vi "CameraSerialPrototype_111.vi"() -> (4 "图像时间戳":u32=16532020 format="%_32g")   [LabVIEW 2015]
uses:
  <vilib>/Instr/_visa.llb/VISA Configure Serial Port (Instr).vi
  MVCAMSDK.dll
  <vilib>/Analysis/NI_AALBase.lvlib
panel:
  out "实时循环时间":u32
  in  "曝光时间":i32=50
  out "平移信号曲线":cluster{"Locations":dbl[], "Amplitudes":dbl[]}[](graph)=[{"Locations"=array[750 elements], "Amplitudes"=array[749 elements]}, {"Locations"=[104.38621227921368, 258.3247060234782, 410.71523318402836, 562.6858730022967, 712.7065754646931], "Amplitudes"=[11153.698204083417, 10559.387052180104, 10974.865031894917, 10500.852817232146, 11059.763900010517]}, {"Locations"=[26.787398227992274, 182.39455189327623, 333.5517219531509, 488.1851999460032, 636.5270621135614], "Amplitudes"=[3284.809720018355, 2039.4564261182056, 3638.2587716464914, 3082.2730888167225, 4217.856016996603]}]
  out "variance 2":dbl caption="方差" format="%0.2f"
  out "光强图 2":dbl[](graph)
  out "variance":dbl caption="方差" format="%0.2f"
  out "光强图":dbl[](graph)
  in  "平移前进":T1=TRUE
  in  "平移计数":u16
  in  "平移一次脉冲数":u16=20
  out "连接的字符串":string
  in  "flow control (0:none)":u16(ring) caption="流控制（0:无）" items=["无", "XON/XOFF", "RTS/CTS", "XON/XOFF & RTS/CTS", "DTR/DSR", "XON/XOFF & DTR/DSR"]
  in  "stop bits (10: 1 bit)":u16=10 caption="停止位（10: 1位）"
  in  "奇偶 (0:none)":enum16{"None", "Odd", "Even", "Mark", "Space"}(ring) caption="奇偶（0:无）"
  in  "数据比特(默认8)":u16(ring)=8 items=["5"=5, "6"=6, "7"=7, "8"=8]
  in  "波特率(默认9600)":u32=9600
  in  "端口":refnum<visa-resource-name>="COM1"
  in  "停止":bool
  out "帧速":u32
  out "帧间耗时\n单位：（0.1ms）":u32
  out "Image":T2(plugin-control)
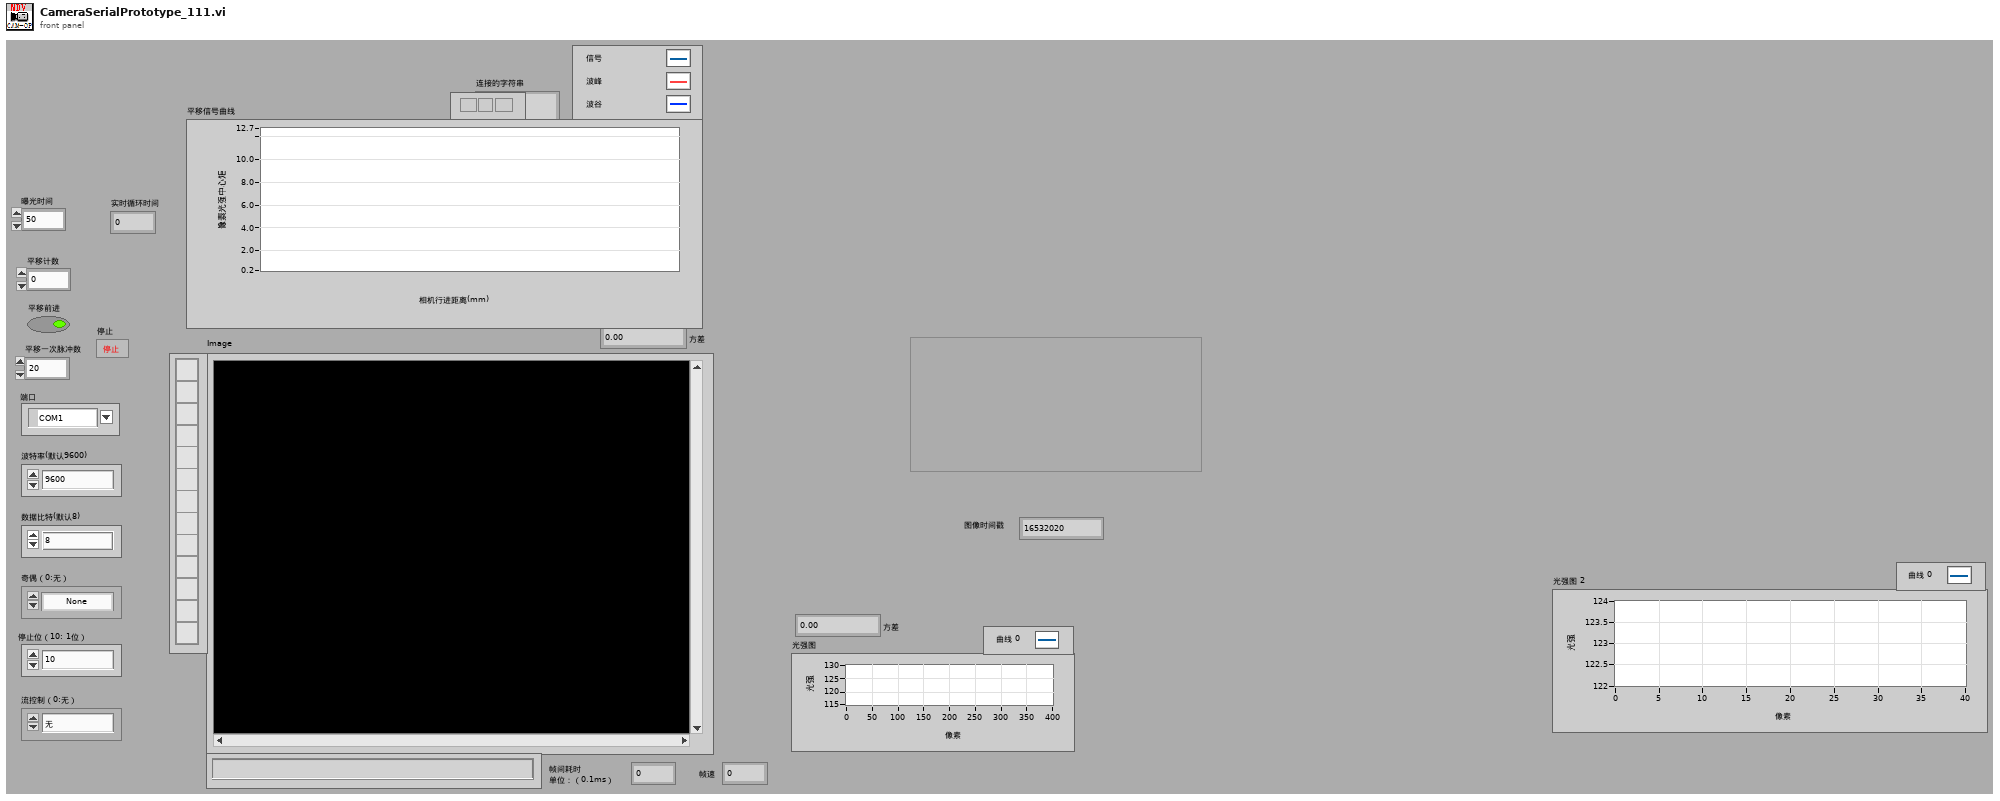
[diagram p1: front panel]
types:
  T1 = typedef "控件 1.ctl" = bool
  T2 = typedef "IMAQ Image.ctl" = refnum<image>
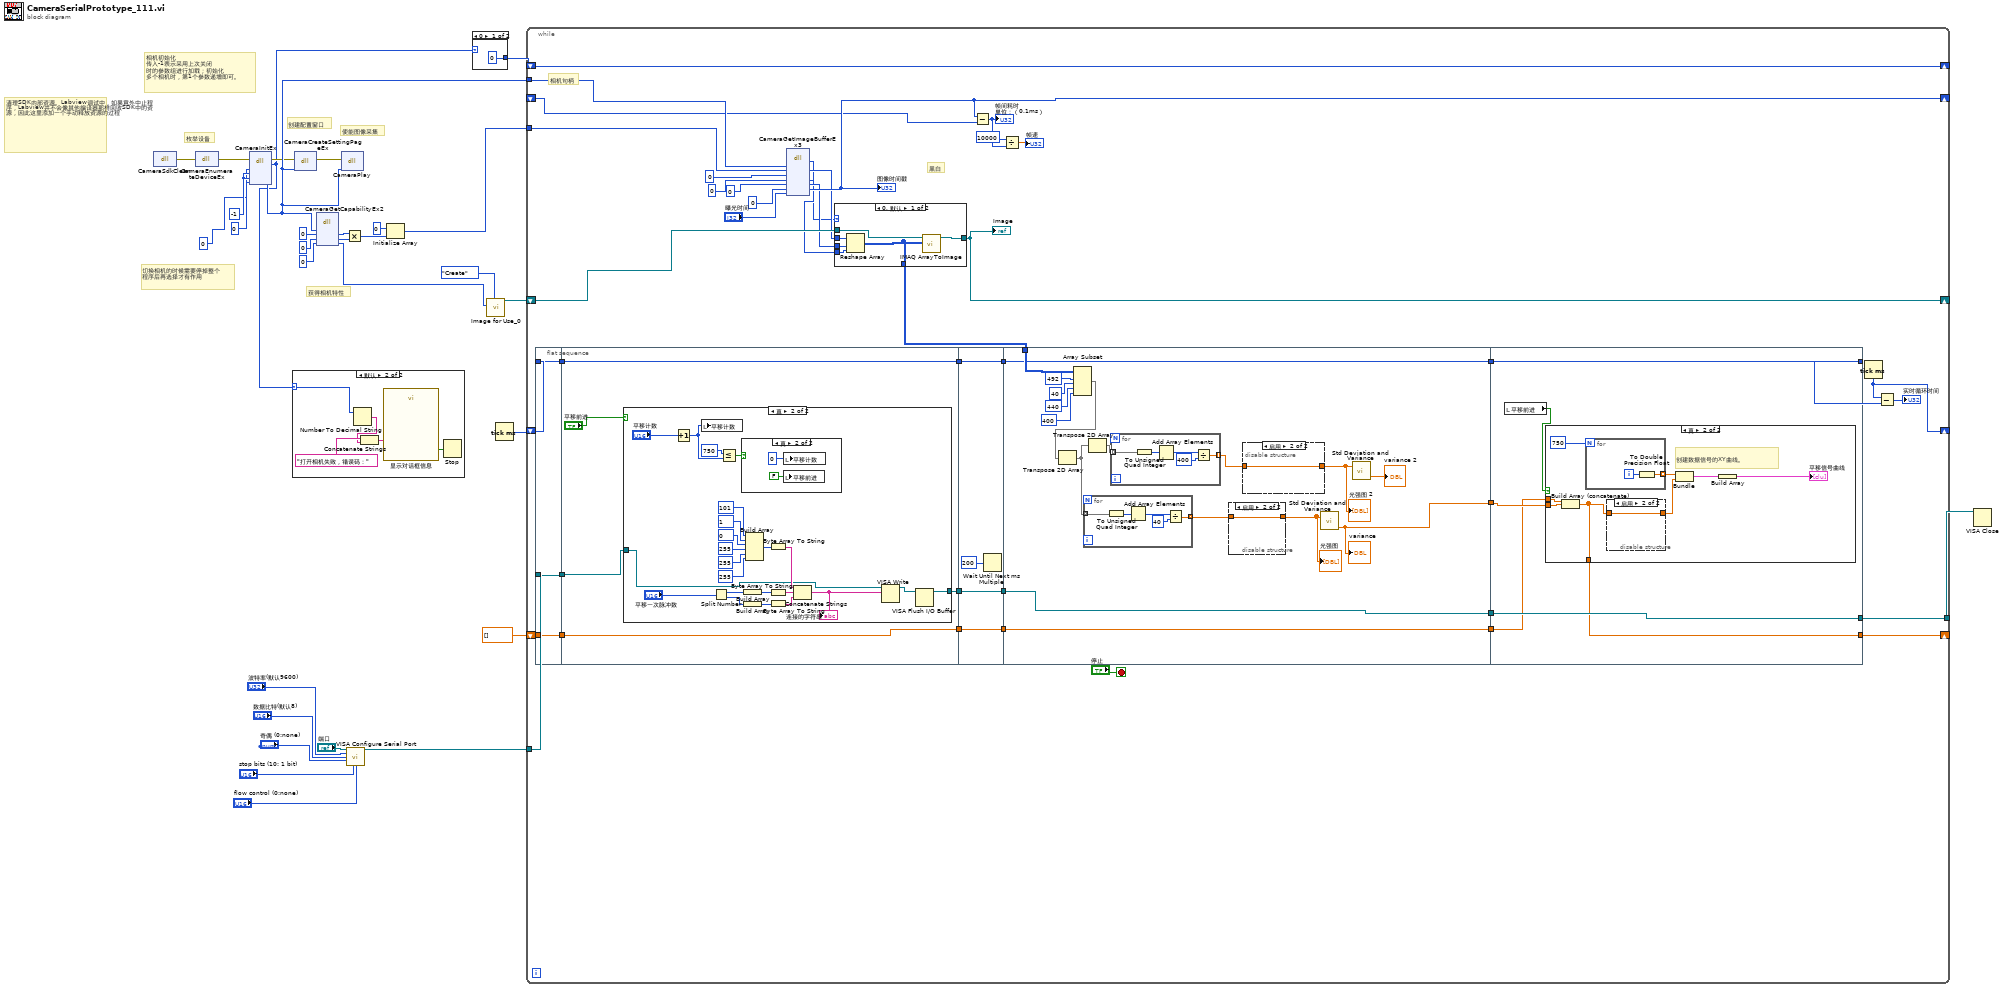
[diagram p0: block diagram]
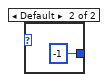
[diagram p2: hidden frame]
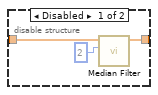
[diagram p6: hidden frame]
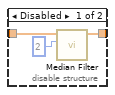
[diagram p7: hidden frame]
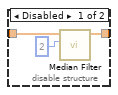
[diagram p9: hidden frame]
diagram:
  w29 = -1
  # "切换相机的时候需要停掉整个\n程序后再选择才有作用"
  # "清理SDK内部资源。Labview调试中，如果意外中止程序，Labview并不会像其他编译器那样回收SDK中的资源，因此这里添加一个手动释放资源的过程"
  # "使能图像采集"
  # "获得相机特性"
  # "创建配置窗口"
  # "相机初始化\n传入-1表示采用上次关闭\n时的参数组进行加载；初始化\n多个相机时，第1个参数递增即可。"
  # "枚举设备"
  n1 = dll-call lib="MVCAMSDK.dll" fn="CameraSdkClean"() -> (error out=w30:errorcluster)  [unwired: 4 in, 1 out]
  n2 = dll-call lib="MVCAMSDK.dll" fn="CameraEnumerateDeviceEx"(error in=w30) -> (error out=w27:errorcluster)  [unwired: 3 in, 1 out]
  n3 = dll-call lib="MVCAMSDK.dll" fn="CameraInitEx"(error in=w27, "相机索引值"=0, "参数加载方式"=w29, "要加载的参数组索引"=w29, "相机句柄"=0) -> (error out=w16:errorcluster, "返回类型"=w14:i32, "相机句柄"=w18:i32)  [unwired: 5 in, 1 out]
  n4 = case shown="默认" w14 {
    selector: w14 -> [_ w35]
    frame 0 {
    }
    frame Default {
      n5 = Number To Decimal String(number=w35) -> (decimal integer string=w32:string)  [unwired: 1 in]
      n6 = Concatenate Strings("打开相机失败，错误码：" ("字符串"), w32) -> (w34:string)
      n7 = call "显示对话框信息"("Message"=w34) -> ("结束"=w36:bool)  [unwired: 9 in, 1 out]
      n8 = Stop(stop? (T)=w36) -> ()
    }
  }
  n9 = dll-call lib="MVCAMSDK.dll" fn="CameraCreateSettingPageEx"(error in=w16, "相机句柄"=w18) -> (error out=w19:errorcluster)  [unwired: 4 in, 1 out]
  n10 = dll-call lib="MVCAMSDK.dll" fn="CameraGetCapabilityEx2"("相机句柄"=w18, "图像最大宽度"=0, "图像最大高度"=0, "是否是彩色相机(返回0:黑白;1:彩色)"=0) -> ("图像最大宽度"=w21:i32, "图像最大高度"=w20:i32, "是否是彩色相机(返回0:黑白;1:彩色)"=w12:i32)  [unwired: 5 in, 2 out]
  n11 = dll-call lib="MVCAMSDK.dll" fn="CameraPlay"(error in=w19, "相机句柄"=w18) -> ()  [unwired: 4 in, 2 out]
  n12 = Multiply(x=w21, y=w20) -> (x*y=w25:i32)
  n13 = call-poly "VISA Configure Serial Port"("VISA resource name"="端口", "baud rate (9600)"="波特率(默认9600)", "data bits (8)"="数据比特(默认8)", "parity (0:none)"="奇偶 (0:none)", "stop bits (10: 1 bit)"="stop bits (10: 1 bit)", "flow control (0:none)"="flow control (0:none)") -> ("VISA resource name out"=w4:refnum<visa-resource-name>)  [unwired: 8 in, 1 out]
  n14 = Initialize Array(0, w25) -> (w17:i32[])
  n15 = case shown="0" w14 {
    tunnel: [0 -1] -> w13
    frame 0 {
    }
    frame Default {
    }
  }
  n16 = call "Image for Use_0.vi"("Command"=enum16{"Create", "Use", "Copy in", "Dispose"}."Create", "Image Type"=w12) -> ("Image out"=w15:T2)  [unwired: 8 in, 1 out]
  n17 = Tick Count (ms)() -> (millisecond timer value=w1:u32)
  n18 = while {
    tunnel: w18 -> [w78]
    tunnel: w17 -> [w80]
    shift-right: [w77] -> _
    shift-left: w13 -> [w77]
    shift-right: [w76] -> _
    shift-left: w15 -> [w79]
    shift-right: [w75] -> _
    shift-left: _ -> [w74]
    tunnel: w4 -> [w53]
    tunnel: [w57] -> w3
    shift-right: [w54] -> _
    shift-left: dbl[] [] -> [w55]
    shift-right: [w49] -> _
    shift-left: w1 -> [w51]
    stop <- "停止" stop-if-true
    # "黑白"
    # "相机句柄"
    n19 = flat-sequence {
      tunnel: w51 -> [w81]
      tunnel: w55 -> [w82]
      tunnel: w53 -> [w83]
      tunnel: [w83] -> w47
      tunnel: [w82] -> w46
      tunnel: [w81] -> w45
      tunnel: [w86] -> w44
      tunnel: [w85] -> w42
      tunnel: w47 -> [w88]
      tunnel: w46 -> [w86]
      tunnel: w45 -> [w85]
      tunnel: [w84] -> w40
      tunnel: w44 -> [w118]
      tunnel: [w118] -> w43
      tunnel: w42 -> [w117]
      tunnel: [w117] -> w41
      tunnel: w40 -> [w116]
      tunnel: [w116] -> w39
      tunnel: w60 -> [w130]
      tunnel: [w122] -> w59
      tunnel: [w119] -> w58
      tunnel: [w121] -> w56
      tunnel: w43 -> [w121]
      tunnel: [w120] -> w52
      tunnel: w41 -> [w120]
      tunnel: w39 -> [w119]
      tunnel: w59 -> [w159]
      tunnel: w58 -> [w158]
      tunnel: [w158] -> w57
      tunnel: w56 -> [w157]
      tunnel: [w156] -> w54
      tunnel: [w154] -> w50
      tunnel: w52 -> [w154]
      frame #0 {
      }
      frame #1 {
        n20 = case shown="真" "平移前进" {
          tunnel: w88 -> [w89 w95]
          tunnel: [w89 w90] -> w84
          frame False {
          }
          frame True {
            n21 = Increment(x="平移计数") -> (x+1=w93:u16)
            n22 = local write "平移计数"(w93) -> ()
            n23 = Split Number(x="平移一次脉冲数") -> (hi(x)=w103:u8, lo(x)=w102:u8)
            n24 = Less Or Equal?(x=750, y=w93) -> (x <= y?=w105:bool)
            n25 = case shown="真" w105 {
              frame False {
              }
              frame True {
                n26 = local write "平移前进"(T1 FALSE ("平移前进")) -> ()
                n27 = local write "平移计数"(u16 0 ("平移计数 2")) -> ()
              }
            }
            n28 = Build Array(w103) -> (w101:u8[])
            n29 = Build Array(w102) -> (w100:u8[])
            n30 = Build Array(101, 1, 0, 255, 255, 255) -> (w99:i32[])
            n31 = Byte Array To String(unsigned byte array=w99) -> (string=w98:string)
            n32 = Byte Array To String(unsigned byte array=w101) -> (string=w97:string)
            n33 = Byte Array To String(unsigned byte array=w100) -> (string=w96:string)
            n34 = Concatenate Strings(w98, w97, w96) -> (w92:string)
            "连接的字符串" <- w92
            n35 = VISA Write(VISA resource name=w95, write buffer=w92) -> (VISA resource name out=w91:refnum<visa-resource-name>)  [unwired: 1 in, 2 out]
            n36 = VISA Flush I/O Buffer(VISA resource name=w91) -> (VISA resource name out=w90:refnum<visa-resource-name>)  [unwired: 2 in, 1 out]
          }
        }
      }
      frame #2 {
        n37 = Wait Until Next ms Multiple(millisecond multiple=u32 200 ("毫秒倍数")) -> ()  [unwired: 1 out]
      }
      frame #3 {
        n38 = Array Subset(array=w130, index (row)=492 ("索引"), length (row)=40 ("长度"), index (col)=440 ("长度"), length (col)=400 ("索引")) -> (w131:u8[][])
        n39 = Transpose 2D Array(2D array=w131) -> (transposed array=w124:u8[][])
        n40 = for {
          tunnel: w124 -> [w148] mode=indexing
          tunnel: [w146] -> w129 mode=indexing
          n41 = To Unsigned Quad Integer(1:w148) -> (0:w147:u64[])
          n42 = Add Array Elements(numeric array=w147) -> (sum=w149:u64)
          n43 = Divide(x=w149, y=u64 40) -> (x/y=w146:dbl)
        }
        n44 = Transpose 2D Array(2D array=w124) -> (transposed array=w125:u8[][])
        n45 = for {
          tunnel: w125 -> [w139] mode=indexing
          tunnel: [w137] -> w123 mode=indexing
          n46 = To Unsigned Quad Integer(1:w139) -> (0:w138:u64[])
          n47 = Add Array Elements(numeric array=w138) -> (sum=w140:u64)
          n48 = Divide(x=w140, y=u64 400) -> (x/y=w137:dbl)
        }
        n49 = disable-structure shown="启用" {
          disable-tunnel: w129 -> [w152 w153]
          disable-tunnel: [w150 w153] -> w128
          frame Disabled {
            n50 = call <vilib>:"Median Filter.vi"("left rank"=2, "X"=w152) -> ("Filtered X"=w150:dbl[])  [unwired: 8 in, 1 out]
          }
          frame Enabled {
          }
        }
        "光强图" <- w128
        n51 = disable-structure shown="启用" {
          disable-tunnel: w123 -> [w143 w144]
          disable-tunnel: [w141 w144] -> w127
          frame Disabled {
            n52 = call <vilib>:"Median Filter.vi"("left rank"=2, "X"=w143) -> ("Filtered X"=w141:dbl[])  [unwired: 8 in, 1 out]
          }
          frame Enabled {
          }
        }
        "光强图 2" <- w127
        n53 = call <vilib>:"Std Deviation and Variance.vi"("X"=w128) -> ("variance"=w122:dbl)  [unwired: 1 in, 2 out]
        "variance" <- w122
        n54 = call <vilib>:"Std Deviation and Variance.vi"("X"=w127) -> ("variance"=→"variance 2":dbl)  [unwired: 1 in, 2 out]
      }
      frame #4 {
        n55 = local read "平移前进"() -> (w155:T1)
        n56 = case shown="真" w155 {
          tunnel: w157 -> [w160 w162]
          tunnel: w159 -> [_ w163]
          tunnel: [w160 w161] -> w156
          frame False {
          }
          frame True {
            # "创建数据信号的XY曲线。"
            n57 = Build Array (concatenate)(w162, w163) -> (w161:dbl[])
            n58 = for {
              N: i64 750 ("数值") -> [_]
              tunnel: [w169] -> w167 mode=indexing
              i -> [w170]
              n59 = To Double Precision Float(number=w170) -> (double precision float=w169:dbl)
            }
            n60 = disable-structure shown="启用" {
              disable-tunnel: w161 -> [w172 w174]
              disable-tunnel: [w171 w174] -> w166
              frame Disabled {
                n61 = call <vilib>:"Median Filter.vi"("left rank"=2, "X"=w172) -> ("Filtered X"=w171:dbl[])  [unwired: 8 in, 1 out]
              }
              frame Enabled {
              }
            }
            n62 = Bundle(w167, w166) -> (w164:cluster{dbl[], dbl[]})  [unwired: 1 in]
            n63 = Build Array(w164) -> (→"平移信号曲线":cluster{dbl[], dbl[]}[])
          }
        }
      }
    }
    n64 = dll-call lib="MVCAMSDK.dll" fn="CameraGetImageBufferEx3"("相机句柄"=w78, "图像数据缓冲区"=w80, "图像输出格式(0:8位灰度;1:24位彩色;2:32位彩色，3：BGR24彩色 4：BGRA32位彩色)"=0, "图像宽度"=0, "图像高度"=0, "时间戳(单位为100微秒)"=0, "抓图超时时间(毫秒)"="曝光时间") -> ("返回类型"=w62:i32, "图像数据缓冲区"=w65:u8[], "图像宽度"=w63:i32, "图像高度"=w64:i32, "时间戳(单位为100微秒)"=w75:u32)  [unwired: 6 in, 2 out]
    "图像时间戳" <- w75
    n65 = case shown="0, 默认" w62 {
      tunnel: w65 -> [w180 _]
      tunnel: w79 -> [w177 w181]
      tunnel: w64 -> [w179 _]
      tunnel: w63 -> [w178 _]
      tunnel: [w176 w181] -> w76
      tunnel: [w175 _] -> w60
      frame 0, Default {
        n66 = Reshape Array(w180, w179, w178) -> (w175:u8[][])
        n67 = call "IMAQ ArrayToImage"("Image Pixels (U8)"=w175, "Image"=w177) -> ("Image Out"=w176:T2)  [unwired: 8 in, 1 out]
      }
      frame -12 {
      }
    }
    "Image" <- w76
    n68 = Subtract(x=w75, y=w74) -> (x-y=w73:u32)
    "帧间耗时\n单位：（0.1ms）" <- w73
    n69 = Divide(x=u32 10000 ("帧间耗时"), y=w73) -> (x/y=→"帧速":dbl)
    n70 = Tick Count (ms)() -> (millisecond timer value=w49:u32)
    n71 = Subtract(x=w49, y=w50) -> (x-y=→"实时循环时间":u32)
  }
  n72 = VISA Close(VISA resource name=w3) -> ()  [unwired: 1 in, 1 out]
